vi "Prompt for Step--Update State Data.vi"(8 "error in (no error)":errorcluster, 9 "Data":variant, 10 "Argument":string, 11 "Image Assertion in":refnum<class "Image Assertion.lvclass">) -> (0 "error out":errorcluster, 3 "Image Assertion out":refnum<class "Image Assertion.lvclass">)   [LabVIEW 2020, in "MacroAssert.lvlib" / "Image Assertion.lvclass"]
doc: "Updates the state data within the \"Prompt for Step\" VI."
uses:
  Image Assertion.lvclass
  Assertion Step/Assertion Step.lvclass
  Image Assertion.lvclass/Image Assertion.ctl
  Image Assertion Type.ctl
  Image Comparator.ctl
  Image Units.ctl
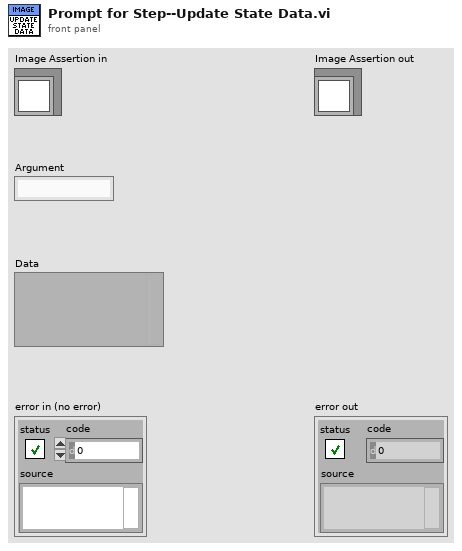
[diagram p1: front panel]
types:
  T1 = typedef "MacroAssert.lvlib/Image Assertion.lvclass/Image Assertion Type.ctl" = enum16{"Control Image", "VI Image", "Window Image", "Cursor Icon"}
  T2 = typedef "MacroAssert.lvlib/Image Assertion.lvclass/Image Comparator.ctl" = enum16{"Equals", "Does not equal"}
  T3 = typedef "MacroAssert.lvlib/Image Assertion.lvclass/Image Units.ctl" = enum16{"Pixels", "Percent"}
  T4 = typedef "imagedata.ctl" = cluster{"image type":i32, "image depth":i32, "image":u8[], "mask":u8[], "colors":u32[], "Rectangle":cluster{"left":i16, "top":i16, "right":i16, "bottom":i16}}
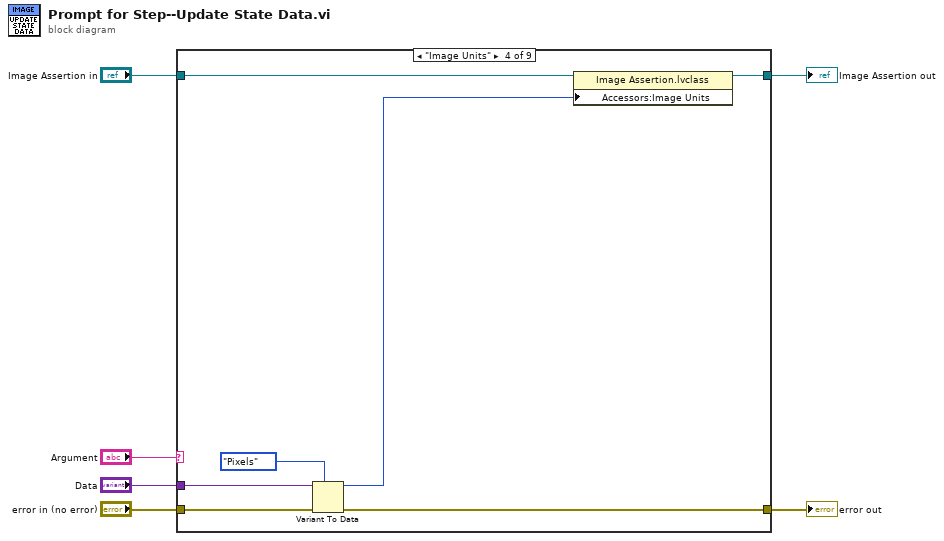
[diagram p0: block diagram]
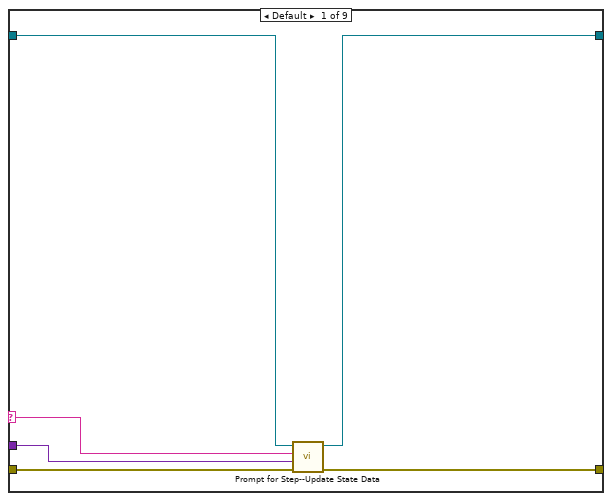
[diagram p2: hidden frame]
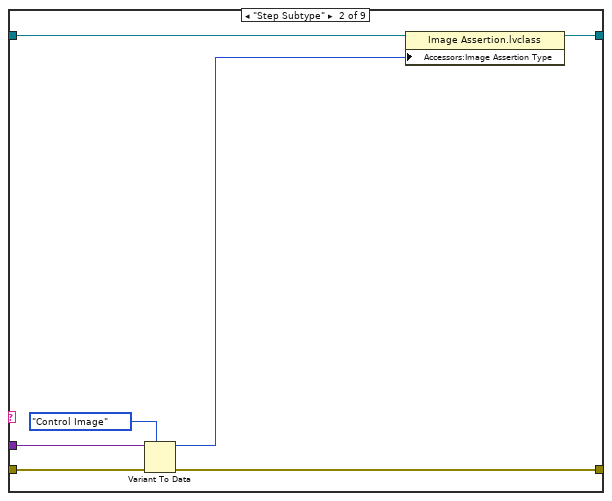
[diagram p3: hidden frame]
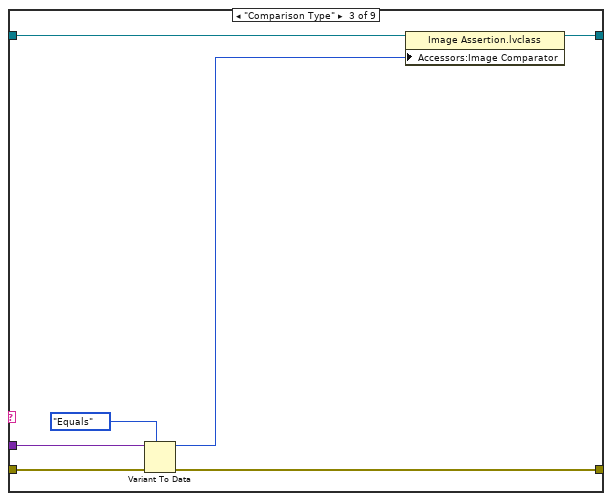
[diagram p4: hidden frame]
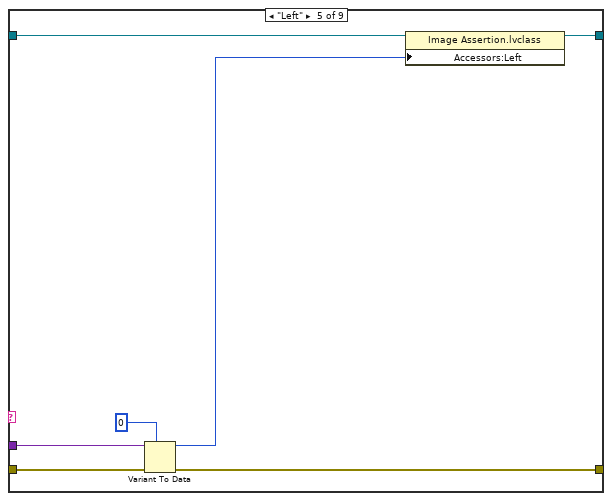
[diagram p5: hidden frame]
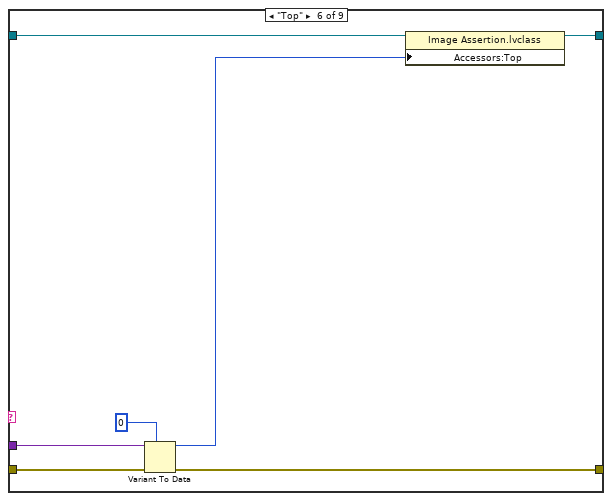
[diagram p6: hidden frame]
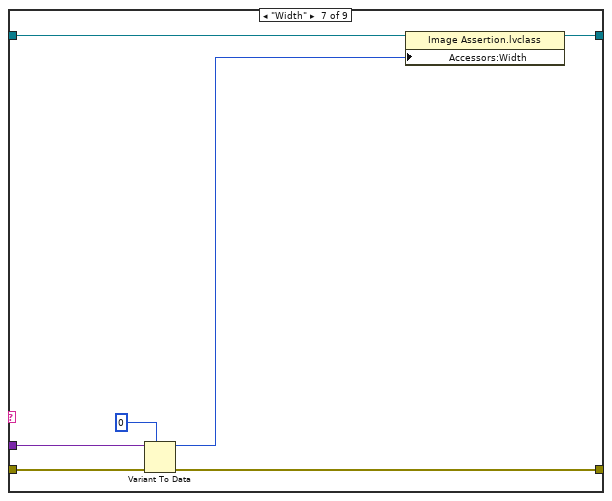
[diagram p7: hidden frame]
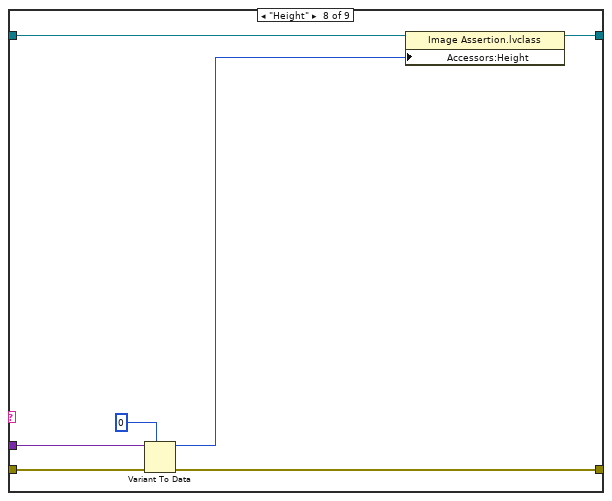
[diagram p8: hidden frame]
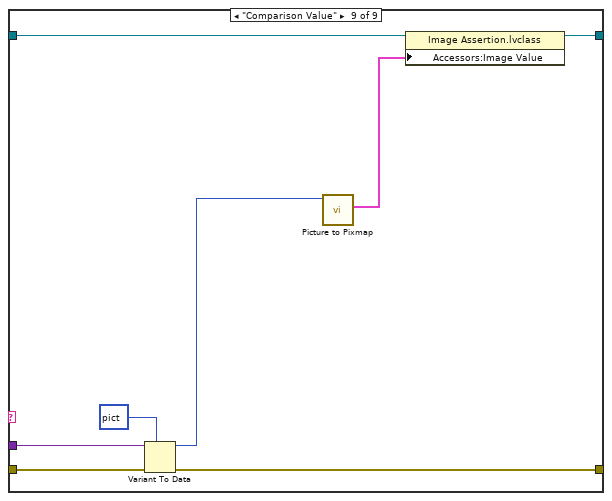
[diagram p9: hidden frame]
diagram:
  n1 = case shown="\"Image Units\"" "Argument" {
    selector: "Argument" -> [w7 _ _ _ _ _ _ _ _]
    tunnel: "Image Assertion in" -> [w10 w19 w26 w33 w40 w47 w54 w61 w69]
    tunnel: "error in (no error)" -> [w12 w17 w24 w31 w38 w45 w52 w59 w67]
    tunnel: [w9 w18 w25 w32 w39 w46 w53 w60 w68] -> w1
    tunnel: [w11 w16 w23 w30 w37 w44 w51 w58 w66] -> w5
    tunnel: "Data" -> [w8 w15 w22 w29 w36 w43 w50 w57 w65]
    frame Default {
      n2 = call-parent "Prompt for Step--Update State Data.vi"("error in (no error)"=w12, "Data"=w8, "Argument"=w7, "Assertion Step in"=w10) -> ("error out"=w11:errorcluster, "Assertion Step out"=w9:refnum<class "Image Assertion.lvclass">)  [unwired: 6 in]
    }
    frame "Step Subtype" {
      n3 = Variant To Data(error in=w17, type=Image_Assertion_Type."Control Image" ("NewVal"), Variant=w15) -> (data=w14:T1, error out=w16:errorcluster)
      n4 = property class="Image Assertion.lvclass"(reference=w19, "Accessors:Image Assertion Type"=w14) -> (reference out=w18:refnum<class "Image Assertion.lvclass">)  [unwired: 1 in, 1 out]
    }
    frame "Comparison Type" {
      n5 = Variant To Data(error in=w24, type=Image_Comparator."Equals" ("NewVal"), Variant=w22) -> (data=w21:T2, error out=w23:errorcluster)
      n6 = property class="Image Assertion.lvclass"(reference=w26, "Accessors:Image Comparator"=w21) -> (reference out=w25:refnum<class "Image Assertion.lvclass">)  [unwired: 1 in, 1 out]
    }
    frame "Image Units" {
      n7 = Variant To Data(error in=w31, type=Image_Units."Pixels" ("NewVal"), Variant=w29) -> (data=w28:T3, error out=w30:errorcluster)
      n8 = property class="Image Assertion.lvclass"(reference=w33, "Accessors:Image Units"=w28) -> (reference out=w32:refnum<class "Image Assertion.lvclass">)  [unwired: 1 in, 1 out]
    }
    frame "Left" {
      n9 = Variant To Data(error in=w38, type=i16 0, Variant=w36) -> (data=w35:i16, error out=w37:errorcluster)
      n10 = property class="Image Assertion.lvclass"(reference=w40, "Accessors:Left"=w35) -> (reference out=w39:refnum<class "Image Assertion.lvclass">)  [unwired: 1 in, 1 out]
    }
    frame "Top" {
      n11 = Variant To Data(error in=w45, type=i16 0, Variant=w43) -> (data=w42:i16, error out=w44:errorcluster)
      n12 = property class="Image Assertion.lvclass"(reference=w47, "Accessors:Top"=w42) -> (reference out=w46:refnum<class "Image Assertion.lvclass">)  [unwired: 1 in, 1 out]
    }
    frame "Width" {
      n13 = Variant To Data(error in=w52, type=i16 0, Variant=w50) -> (data=w49:i16, error out=w51:errorcluster)
      n14 = property class="Image Assertion.lvclass"(reference=w54, "Accessors:Width"=w49) -> (reference out=w53:refnum<class "Image Assertion.lvclass">)  [unwired: 1 in, 1 out]
    }
    frame "Height" {
      n15 = Variant To Data(error in=w59, type=i16 0, Variant=w57) -> (data=w56:i16, error out=w58:errorcluster)
      n16 = property class="Image Assertion.lvclass"(reference=w61, "Accessors:Height"=w56) -> (reference out=w60:refnum<class "Image Assertion.lvclass">)  [unwired: 1 in, 1 out]
    }
    frame "Comparison Value" {
      n17 = Variant To Data(error in=w67, type=picture data[5B] ("picture"), Variant=w65) -> (data=w63:picture, error out=w66:errorcluster)
      n18 = call <vilib>:"Picture to Pixmap.vi"("picture"=w63) -> ("image data"=w62:T4)  [unwired: 9 in, 1 out]
      n19 = property class="Image Assertion.lvclass"(reference=w69, "Accessors:Image Value"=w62) -> (reference out=w68:refnum<class "Image Assertion.lvclass">)  [unwired: 1 in, 1 out]
    }
  }
  "error out" <- w5
  "Image Assertion out" <- w1
